vi "Camera-Device2Cluster.vi"(1 "uSerialNumber IN":u32, 2 "Error IN":errorcluster, 3 "hCamera IN":u32) -> (0 "Camera Device OUT":T1)   [LabVIEW 2010]
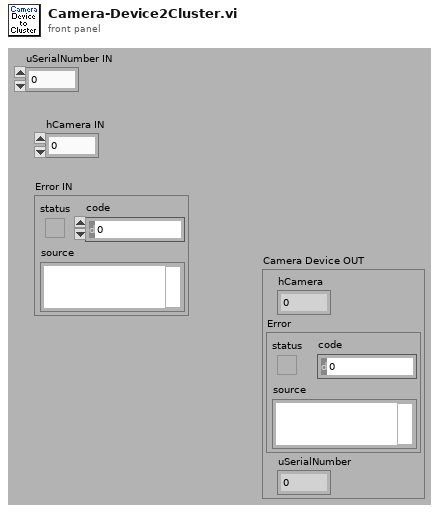
[diagram p1: front panel]
types:
  T1 = cluster{"hCamera":u32, "Error":errorcluster, "uSerialNumber":u32}
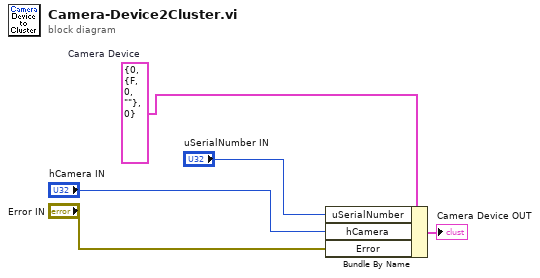
[diagram p0: block diagram]
diagram:
  w3 = T1 {"hCamera"=0, "Error"={"status"=FALSE, "code"=0, "source"=""}, "uSerialNumber"=0}  # Camera Device
  n1 = Bundle By Name(cluster=w3, "uSerialNumber"="uSerialNumber IN", "hCamera"="hCamera IN", "Error"="Error IN") -> (→"Camera Device OUT":T1)
